vi "Write_RobotMode.vi"(8 "error in (no error)":errorcluster, 10 "RobotMode":enum16{"Auto", "Teleop", "Disabled"}(ring), 11 "RobotSubsystem in":refnum<class "RobotSubsystem.lvclass">) -> (0 "error out":errorcluster, 3 "RobotSubsystem out":refnum<class "RobotSubsystem.lvclass">)   [LabVIEW 2017, in "RobotSubsystem.lvclass"]
uses:
  RobotSubsystem.lvclass
  RobotSubsystem.lvclass/RobotSubsystem.ctl
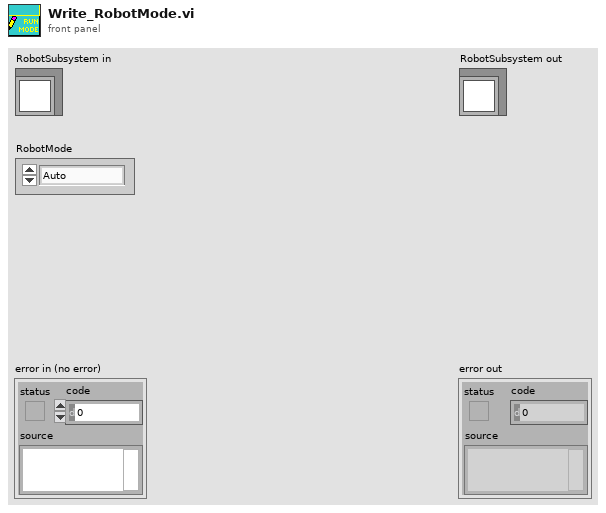
[diagram p1: front panel]
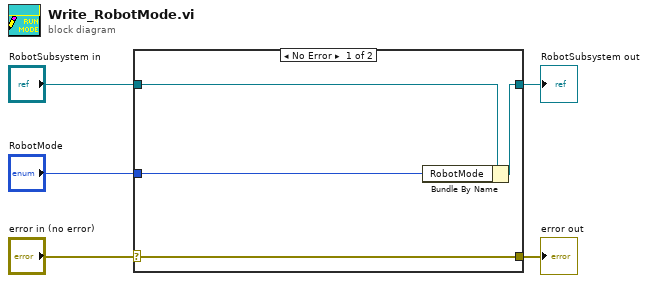
[diagram p0: block diagram]
diagram:
  n1 = case shown="No Error" "error in (no error)" {
    selector: "error in (no error)" -> [w9 w10]
    tunnel: [w9 w10] -> w4
    tunnel: [w7 w11] -> w2
    tunnel: "RobotSubsystem in" -> [w8 w11]
    tunnel: "RobotMode" -> [w6 _]
    frame No Error {
      n2 = Bundle By Name(cluster=w8, "RobotMode"=w6) -> (w7:refnum<class "RobotSubsystem.lvclass">)
    }
    frame Error {
    }
  }
  "error out" <- w4
  "RobotSubsystem out" <- w2
